vi "Omron Serial FINS-Response Data.vi"(8 "error in":errorcluster, 11 "Buffer Data In":T1={"VISA Resource Name"="", "Wait For Read(ms)"=50, "Command Code"=enum."Memory area read", "Command String"="", "Read Bytes"=0, "Response String"=""}) -> (0 "error out":errorcluster, 2 "Data":i16[](array[numeric]), 3 "Buffer Data Out":T1={"VISA Resource Name"="", "Wait For Read(ms)"=50, "Command Code"=enum."Memory area read", "Command String"="", "Read Bytes"=0, "Response String"=""})   [LabVIEW 2016]
uses:
  Data Def/Omron Serial FINS-Buffer Data.ctl
  Data Def/Omron Serial FINS-Command Code.ctl
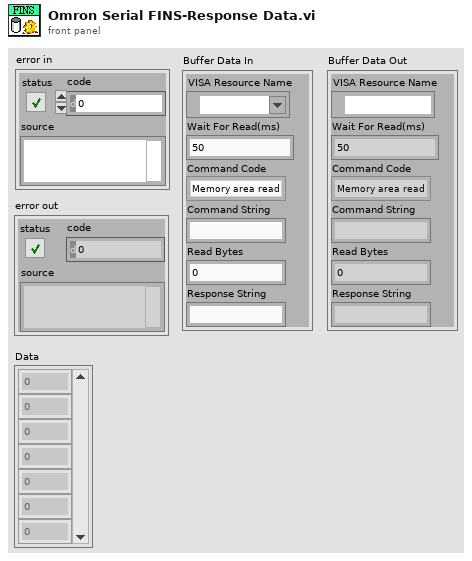
[diagram p1: front panel]
types:
  T1 = typedef "Omron Serial FINS-Buffer Data.ctl" = cluster{"VISA Resource Name":refnum<visa-resource-name>, "Wait For Read(ms)":u32, "Command Code":T2, "Command String":string, "Read Bytes":u32, "Response String":string}
  T2 = typedef "Omron Serial FINS-Command Code.ctl" = enum16{"Memory area read", "Memory area write"}
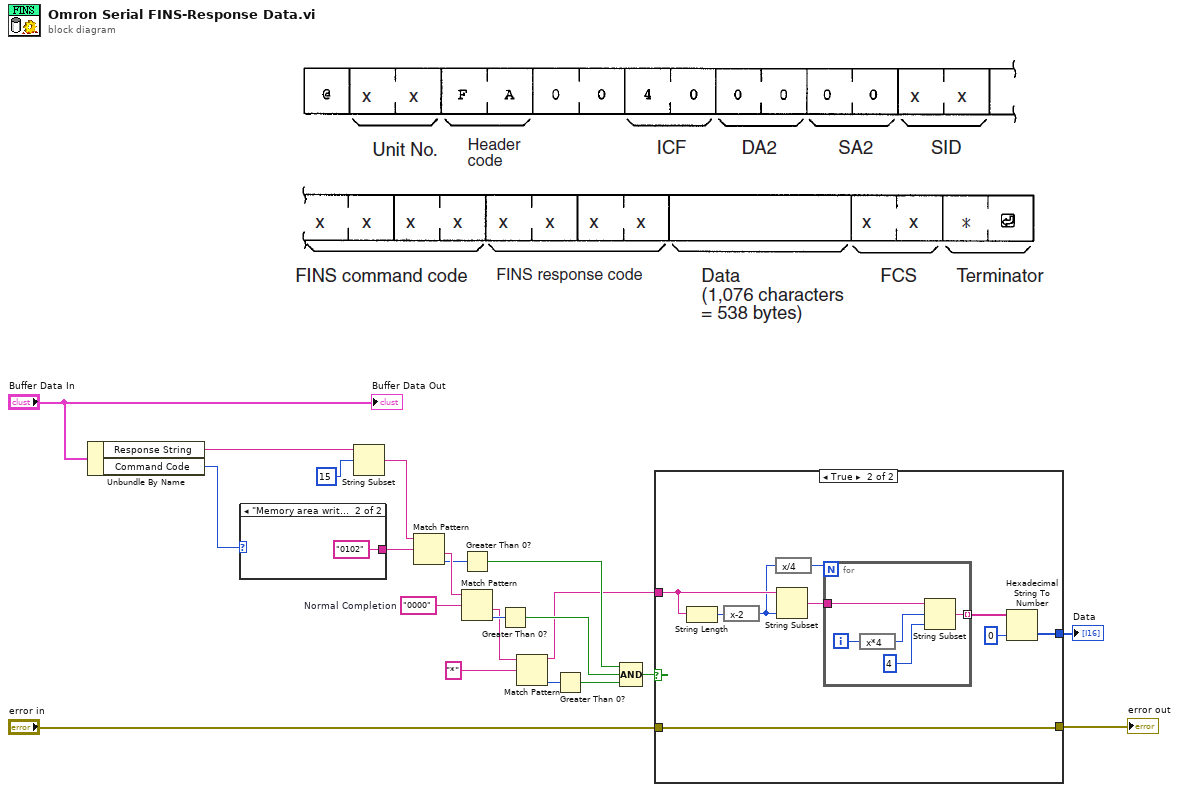
[diagram p0: block diagram]
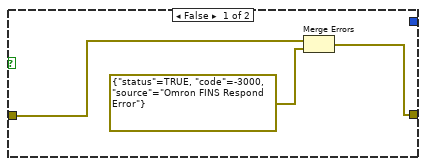
[diagram p2: hidden frame]
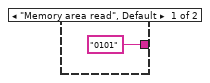
[diagram p3: hidden frame]
diagram:
  w18 = "0000"  # Normal Completion
  n1 = Unbundle By Name("Buffer Data In") -> ("Response String"=w3:string, "Command Code"=w2:T2)
  n2 = case shown="\"Memory area write\"" w2 {
    tunnel: ["0101" ("Command code") "0102" ("Command code")] -> w20
    frame "Memory area read", Default {
    }
    frame "Memory area write" {
    }
  }
  n3 = String Subset(string=w3, offset (0)=15) -> (substring=w19:string)  [unwired: 1 in]
  n4 = Match Pattern(string=w19, regular expression=w20) -> (after substring=w17:string, offset past match=w16:i32)  [unwired: 1 in, 2 out]
  n5 = Greater Than 0?(x=w16) -> (x > 0?=w9:bool)
  n6 = Match Pattern(string=w17, regular expression=w18) -> (after substring=w13:string, offset past match=w15:i32)  [unwired: 1 in, 2 out]
  n7 = Greater Than 0?(x=w15) -> (x > 0?=w10:bool)
  n8 = Match Pattern(string=w13, regular expression="*") -> (before substring=w7:string, offset past match=w12:i32)  [unwired: 1 in, 2 out]
  n9 = Greater Than 0?(x=w12) -> (x > 0?=w11:bool)
  n10 = Compound Arithmetic op=AND(w9, w10, w11) -> (w8:bool)
  n11 = case shown="True" w8 {
    tunnel: w7 -> [_ w34]
    tunnel: [_ w28] -> w5
    tunnel: "error in" -> [w26 w27]
    tunnel: [w25 w27] -> w4
    frame False {
      n12 = Merge Errors(w26, errorcluster {"status"=TRUE, "code"=-3000, "source"="Omron FINS Respond Error"} ("error in")) -> (w25:errorcluster)
    }
    frame True {
      n13 = String Length(string=w34) -> (length=w35:i32)
      n14 = expression code="x-2"(w35) -> (w32:i32)
      n15 = expression code="x/4"(w32) -> (w31:i32)
      n16 = String Subset(string=w34, length (rest)=w32) -> (substring=w33:string)  [unwired: 1 in]
      n17 = for {
        N: w31 -> [_]
        tunnel: w33 -> [w40]
        tunnel: [w36] -> w30 mode=indexing
        i -> [w38]
        n18 = expression code="x*4"(w38) -> (w37:i32)
        n19 = String Subset(string=w40, offset (0)=w37, length (rest)=4 ("length (rest)")) -> (substring=w36:string)
      }
      n20 = Hexadecimal String To Number(string=w30, default (0uL)=i16 0 ("default (0 U32)")) -> (number=w28:i16[])  [unwired: 1 in, 1 out]
    }
  }
  "error out" <- w4
  "Data" <- w5
  "Buffer Data Out" <- "Buffer Data In"
